vi "Obtain Request Events.vi"(8 "error in (no error)":errorcluster, 10 "Create New?":bool) -> (0 "error out":errorcluster, 2 "MQTTClient Request Events":T1)   [LabVIEW 2024, in "MQTTClient.lvlib"]
doc: "This VI Obtains/Creates the Requests events that will be used for other modules to communicate with the module that owns this VI. These Requests events will be accessed only via Public API methods for this module.\n\n<b>NOTE</b>: The contents of this VI are automatically generated and modified by the <b>Tools > Delacor > DQMH</b> utilities. Consider using those utilities instead of making your own modifications to this VI.\n_____\nBased on Delacor QMH Project Template 3.1.0.34."
uses:
  MQTTClient.lvlib
  Request Events--cluster.ctl
  Stop Argument--cluster.ctl
  Show Panel Argument--cluster.ctl
  Hide Panel Argument--cluster.ctl
  Get Module Execution Status Argument--cluster.ctl
  Show Diagram Argument--cluster.ctl
  Change Panel Argument--cluster.ctl
  <vilib>/MGI/Panel Manager/Panel/Panel/Panel.lvclass
  Initialise Connection Argument--cluster.ctl
  Ping Connection Argument--cluster.ctl
  Publish to MQTT Topic Argument--cluster.ctl
  Close Connection Argument--cluster.ctl
  Connect to MQTT Server Argument--cluster.ctl
  Reset Ping Helper Loop Timeout Argument--cluster.ctl
  Sleep Ping Helper Loop Argument--cluster.ctl
  Register MQTT Client Events Argument--cluster.ctl
  <vilib>/LabVIEW Open Source Project/MQTT Client/Client class/Public Events -- cluster.ctl
  <vilib>/LabVIEW Open Source Project/MQTT Control Packets/Control Packets/CONNACK/Connect Return Code -- enum.ctl
  <vilib>/LabVIEW Open Source Project/MQTT Control Packets/Control Packets/PUBLISH/PUBLISH.lvclass
  <vilib>/LabVIEW Open Source Project/MQTT Connection/MQTT_Base/Base Class/Public Events -- cluster.ctl
  Subscribe to MQTT Topic Argument--cluster.ctl
  Launch Argument--cluster.ctl
  Wake Connection Helper Loop Argument--cluster.ctl
  <vilib>/LabVIEW Open Source Project/MQTT Connection/MQTT_Base/Base Class/MQTT_Base.lvclass
  <vilib>/LabVIEW Open Source Project/MQTT Control Packets/Control Packets/CONNACK/CONNACK.lvclass
  <vilib>/LabVIEW Open Source Project/MQTT Client/Client class/Client.lvclass
panel:
  # "NOTE: The contents of this VI are automatically generated and modified by the Tools > Delacor > DQMH utilities. Consider using those utilities instead of making your own modifications to this VI."
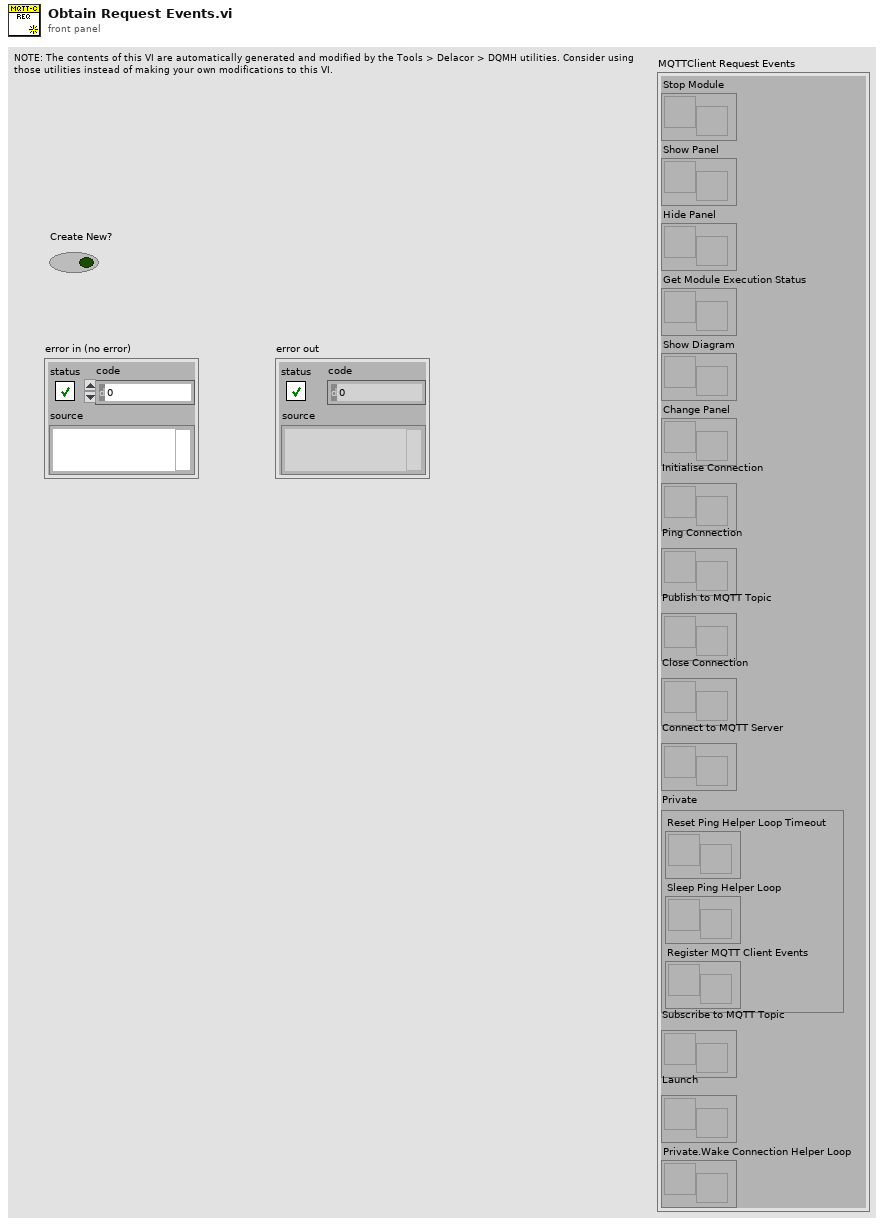
[diagram p1: front panel]
types:
  T1 = typedef "MQTTClient.lvlib/Request Events--cluster.ctl" = cluster{"Stop Module":refnum<user-event>, "Show Panel":refnum<user-event>, "Hide Panel":refnum<user-event>, "Get Module Execution Status":refnum<user-event>, "Show Diagram":refnum<user-event>, "Change Panel":refnum<user-event>, "Initialise Connection":refnum<user-event>, "Ping Connection":refnum<user-event>, "Publish to MQTT Topic":refnum<user-event>, "Close Connection":refnum<user-event>, "Connect to MQTT Server":refnum<user-event>, "Private":cluster{"Reset Ping Helper Loop Timeout":refnum<user-event>, "Sleep Ping Helper Loop":refnum<user-event>, "Register MQTT Client Events":refnum<user-event>}, "Subscribe to MQTT Topic":refnum<user-event>, "Launch":refnum<user-event>, "Private.Wake Connection Helper Loop":refnum<user-event>}
  T2 = typedef "MQTTClient.lvlib/Wake Connection Helper Loop Argument--cluster.ctl" = cluster{"Boolean":bool}
  T3 = typedef "MQTTClient.lvlib/Launch Argument--cluster.ctl" = cluster{"Boolean":bool}
  T4 = typedef "MQTTClient.lvlib/Register MQTT Client Events Argument--cluster.ctl" = cluster{"Client Public Events":T5, "MQTT Public Events":T6}
  T5 = typedef "MQTT Client.lvlib/Client.lvclass/Public Events -- cluster.ctl" = cluster{"Connection Status":refnum<user-event>, "Connected":refnum<user-event>, "Application Message":refnum<user-event>}
  T6 = typedef "MQTT Base.lvlib/MQTT_Base.lvclass/Public Events -- cluster.ctl" = cluster{"Stop Event":refnum<user-event>, "Error Event":refnum<user-event>, "Inbound Message":refnum<user-event>}
  T7 = typedef "MQTTClient.lvlib/Subscribe to MQTT Topic Argument--cluster.ctl" = cluster{"Topic":string}
  T8 = typedef "MQTTClient.lvlib/Sleep Ping Helper Loop Argument--cluster.ctl" = cluster{"Boolean":bool}
  T9 = typedef "MQTTClient.lvlib/Reset Ping Helper Loop Timeout Argument--cluster.ctl" = cluster{"Boolean":bool}
  T10 = typedef "MQTTClient.lvlib/Connect to MQTT Server Argument--cluster.ctl" = cluster{"Boolean":bool}
  T11 = typedef "MQTTClient.lvlib/Close Connection Argument--cluster.ctl" = cluster{"Boolean":bool}
  T12 = typedef "MQTTClient.lvlib/Publish to MQTT Topic Argument--cluster.ctl" = cluster{"Topic":string, "Value":string}
  T13 = typedef "MQTTClient.lvlib/Ping Connection Argument--cluster.ctl" = cluster{"Boolean":bool}
  T14 = typedef "MQTTClient.lvlib/Initialise Connection Argument--cluster.ctl" = cluster{"Client ID":string, "Server Address":string, "Server Port":u16}
  T15 = typedef "MQTTClient.lvlib/Change Panel Argument--cluster.ctl" = cluster{"New Panel":refnum<class "Panel.lvclass">}
  T16 = typedef "MQTTClient.lvlib/Hide Panel Argument--cluster.ctl" = cluster{"Hide Panel?":bool}
  T17 = typedef "MQTTClient.lvlib/Show Panel Argument--cluster.ctl" = cluster{"Show Panel?":bool}
  T18 = typedef "MQTTClient.lvlib/Show Diagram Argument--cluster.ctl" = cluster{"Debug?":bool}
  T19 = typedef "MQTTClient.lvlib/Get Module Execution Status Argument--cluster.ctl" = cluster{"Running?":bool}
  T20 = typedef "MQTTClient.lvlib/Stop Argument--cluster.ctl" = cluster{"Origin":string, "Exit via Stop Module Req?":bool, "Wait for Module to stop?":bool}
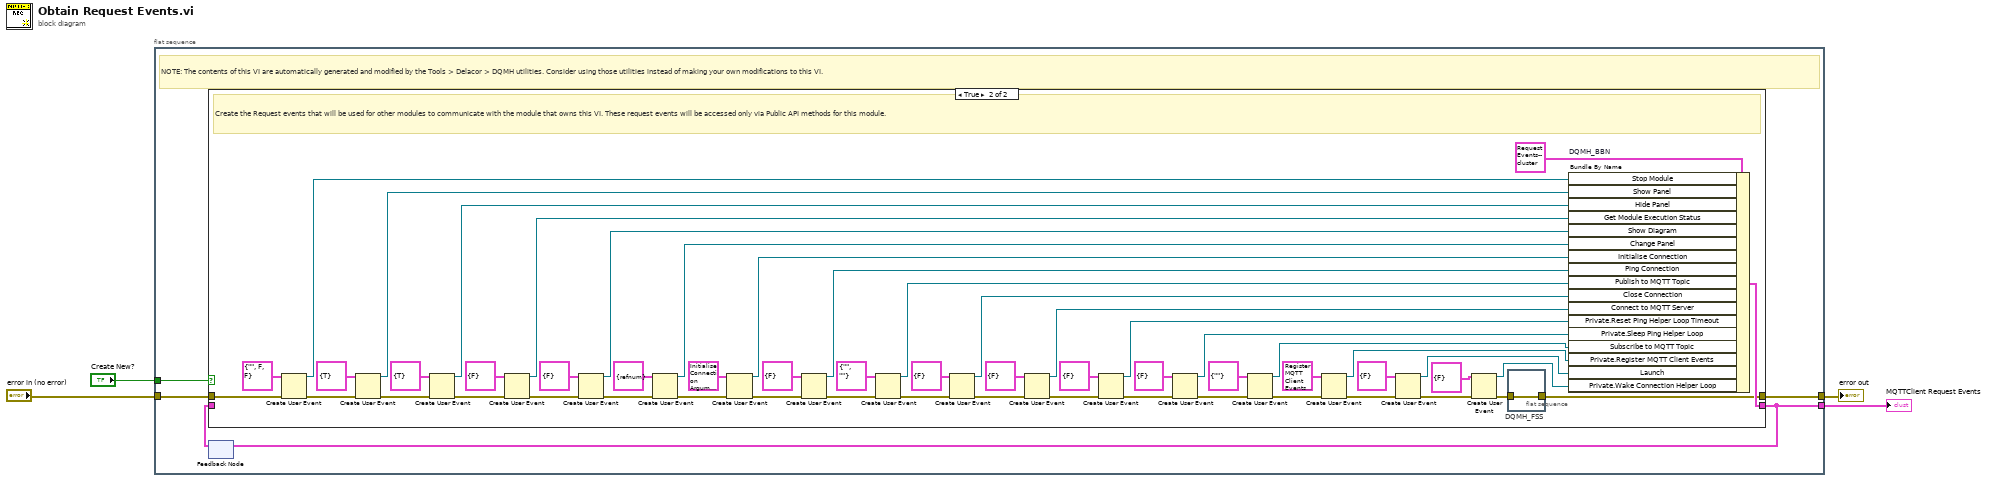
[diagram p0: block diagram]
diagram:
  n1 = flat-sequence {
    tunnel: [w9] -> w4
    tunnel: "error in (no error)" -> [w8]
    tunnel: [w6] -> w2
    tunnel: "Create New?" -> [w5]
    frame #0 {
      # "NOTE: The contents of this VI are automatically generated and modified by the Tools > Delacor > DQMH utilities. Consider using those utilities instead of making your own modifications to this VI."
      n2 = feedback #1() -> (w7:T1)  [unwired: 1 in]
      n3 = case shown="True" w5 {
        tunnel: [w10 w56] -> w9
        tunnel: w8 -> [w10 w66]
        tunnel: [w11 w63] -> w6
        tunnel: w7 -> [w11 _]
        frame False {
          # "Obtain the Request events that were created in a previous call to this VI."
        }
        frame True {
          # "Create the Request events that will be used for other modules to communicate with the module that owns this VI. These request events will be accessed only via Public API methods for this module."
          n4 = Create User Event(user event datatype=T20 {"Origin"="", "Exit via Stop Module Req?"=FALSE, "Wait for Module to stop?"=FALSE} ("Stop Argument"), error in=w66) -> (user event=w64:refnum<user-event>, error out=w61:errorcluster)
          n5 = Create User Event(user event datatype=T17 {"Show Panel?"=TRUE} ("Show Panel Argument"), error in=w61) -> (user event=w60:refnum<user-event>, error out=w59:errorcluster)
          n6 = Create User Event(user event datatype=T16 {"Hide Panel?"=TRUE} ("Hide Panel Argument"), error in=w59) -> (user event=w58:refnum<user-event>, error out=w57:errorcluster)
          n7 = Create User Event(user event datatype=T19 {"Running?"=FALSE} ("Get Module Execution Status Argument"), error in=w57) -> (user event=w54:refnum<user-event>, error out=w55:errorcluster)
          n8 = Create User Event(user event datatype=T18 {"Debug?"=FALSE} ("Show Diagram Argument"), error in=w55) -> (user event=w51:refnum<user-event>, error out=w52:errorcluster)
          n9 = Create User Event(user event datatype=T15 {"New Panel"=refnum} ("Change Panel Argument"), error in=w52) -> (user event=w46:refnum<user-event>, error out=w47:errorcluster)
          n10 = Create User Event(user event datatype=T14 {"Client ID"="BTSCLIENT-001", "Server Address"="localhost", "Server Port"=1883} ("Initialise Connection Argument"), error in=w47) -> (user event=w43:refnum<user-event>, error out=w44:errorcluster)
          n11 = Create User Event(user event datatype=T13 {"Boolean"=FALSE} ("Ping Connection Argument"), error in=w44) -> (user event=w40:refnum<user-event>, error out=w41:errorcluster)
          n12 = Create User Event(user event datatype=T12 {"Topic"="", "Value"=""} ("Publish to MQTT Topic Argument"), error in=w41) -> (user event=w37:refnum<user-event>, error out=w38:errorcluster)
          n13 = Create User Event(user event datatype=T11 {"Boolean"=FALSE} ("Close Connection Argument"), error in=w38) -> (user event=w34:refnum<user-event>, error out=w35:errorcluster)
          n14 = Create User Event(user event datatype=T10 {"Boolean"=FALSE} ("Connect to MQTT Server Argument"), error in=w35) -> (user event=w31:refnum<user-event>, error out=w32:errorcluster)
          n15 = Create User Event(user event datatype=T9 {"Boolean"=FALSE} ("Reset Ping Helper Loop Timeout Argument"), error in=w32) -> (user event=w28:refnum<user-event>, error out=w29:errorcluster)
          n16 = Create User Event(user event datatype=T8 {"Boolean"=FALSE} ("Sleep Ping Helper Loop Argument"), error in=w29) -> (user event=w25:refnum<user-event>, error out=w26:errorcluster)
          n17 = Create User Event(user event datatype=T7 {"Topic"=""} ("Subscribe to MQTT Topic Argument"), error in=w26) -> (user event=w22:refnum<user-event>, error out=w23:errorcluster)
          n18 = Create User Event(user event datatype=T4 {"Client Public Events"={"Connection Status"=refnum, "Connected"=refnum, "Application Message"=refnum}, "MQTT Public Events"={"Stop Event"=refnum, "Error Event"=refnum, "Inbound Message"=refnum}} ("Register MQTT Client Events Argument"), error in=w23) -> (user event=w19:refnum<user-event>, error out=w20:errorcluster)
          n19 = Create User Event(user event datatype=T3 {"Boolean"=FALSE} ("Launch Argument"), error in=w20) -> (user event=w16:refnum<user-event>, error out=w17:errorcluster)
          n20 = Create User Event(user event datatype=T2 {"Boolean"=FALSE} ("Wake Connection Helper Loop Argument"), error in=w17) -> (user event=w13:refnum<user-event>, error out=w14:errorcluster)
          n21 = flat-sequence "DQMH_FSS" {
            tunnel: w14 -> [w67]
            tunnel: [w67] -> w56
            frame #0 {
            }
          }
          n22 = Bundle By Name "DQMH_BBN"(cluster=T1 {"Stop Module"=refnum, "Show Panel"=refnum, "Hide Panel"=refnum, "Get Module Execution Status"=refnum, "Show Diagram"=refnum, "Change Panel"=refnum, "Initialise Connection"=refnum, "Ping Connection"=refnum, "Publish to MQTT Topic"=refnum, "Close Connection"=refnum, "Connect to MQTT Server"=refnum, "Private"={"Reset Ping Helper Loop Timeout"=refnum, "Sleep Ping Helper Loop"=refnum, "Register MQTT Client Events"=refnum}, "Subscribe to MQTT Topic"=refnum, "Launch"=refnum, "Private.Wake Connection Helper Loop"=refnum} ("output cluster"), "Stop Module"=w64, "Show Panel"=w60, "Hide Panel"=w58, "Get Module Execution Status"=w54, "Show Diagram"=w51, "Change Panel"=w46, "Initialise Connection"=w43, "Ping Connection"=w40, "Publish to MQTT Topic"=w37, "Close Connection"=w34, "Connect to MQTT Server"=w31, "Private.Reset Ping Helper Loop Timeout"=w28, "Private.Sleep Ping Helper Loop"=w25, "Subscribe to MQTT Topic"=w22, "Private.Register MQTT Client Events"=w19, "Launch"=w16, "Private.Wake Connection Helper Loop"=w13) -> (w63:T1)
        }
      }
      n23 = feedback-in #1(w6) -> ()
    }
  }
  "MQTTClient Request Events" <- w2
  "error out" <- w4
